vi "Variant to JSON.vi"(8 "error in (no error)":errorcluster, 9 "Pretty Print? (F)":bool, 10 "Enums as string? (F)":bool, 11 "Variant in":variant) -> (0 "error out":errorcluster, 3 "JSON":string)   [LabVIEW 2019, in "labview_json.lvlib"]
doc: "Exports a <b>Variant</b> to a <b>JSON</b> string. Set <b>Enums as string?</b> to True to export enums as a string, otherwise enums are considered unsigned integers. Set <b>Pretty Print?</b> to True to add indentation to the output JSON string.\nCreated by: Ryan Pacini"
uses:
  labview_json.lvlib
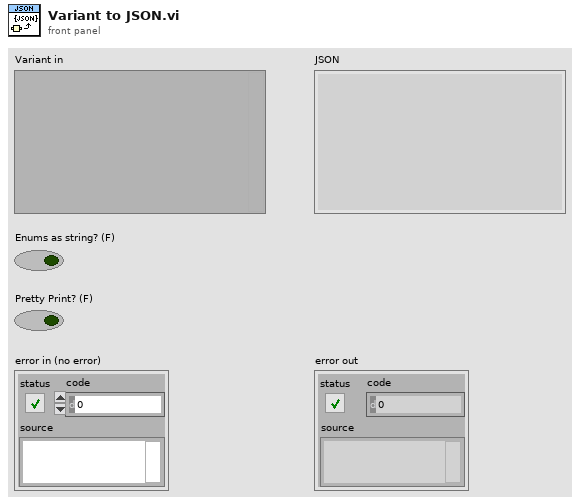
[diagram p1: front panel]
types:
  T1 = typedef "labview_json.lvlib/Element.ctl" = cluster{"Key":string, "Type":T2, "Value":variant, "IsRootPath":bool}
  T2 = typedef "labview_json.lvlib/Element Type.ctl" = enum8{"NULL", "OBJECT", "ARRAY", "BOOL", "INT", "UINT", "FLOAT", "STRING"}
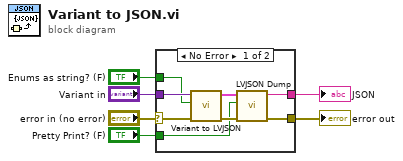
[diagram p0: block diagram]
diagram:
  n1 = case shown="No Error" "error in (no error)" {
    selector: "error in (no error)" -> [w14 w15]
    tunnel: "Variant in" -> [w13 _]
    tunnel: [w9 w15] -> w4
    tunnel: "Enums as string? (F)" -> [w12 _]
    tunnel: [w8 _] -> w2
    tunnel: "Pretty Print? (F)" -> [w7 _]
    frame No Error {
      n2 = call "Variant to LVJSON.vi"("error in (no error)"=w14, "Enums as string? (F)"=w12, "Variant in"=w13) -> ("error out"=w11:errorcluster, "Element out"=w10:T1)  [unwired: 7 in]
      n3 = call "LVJSON Dump.vi"("error in (no error)"=w11, "Pretty Print? (F)"=w7, "Root Element in"=w10) -> ("error out"=w9:errorcluster, "JSON out"=w8:string)  [unwired: 6 in, 1 out]
    }
    frame Error {
    }
  }
  "error out" <- w4
  "JSON" <- w2
